vi "FPGA_target_reset_memory.vi"(0 "mem_addr_in":u32) -> (14 "mem_addr_out":u32)   [LabVIEW 2014]
doc: "Clears memory from specified index."
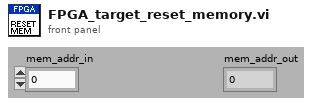
[diagram p1: front panel]
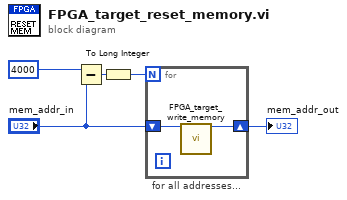
[diagram p0: block diagram]
diagram:
  n1 = Subtract(x=u32 4000, y="mem_addr_in") -> (x-y=w3:u32)
  n2 = To Long Integer(number=w3) -> (32bit integer=w4:i32)
  n3 = for "for all addresses..." {
    N: w4 -> [_]
    shift-right: [w6] -> w1
    shift-left: "mem_addr_in" -> [w7]
    n4 = call "FPGA_target_write_memory.vi"("mem_addr_in"=w7) -> ("mem_addr_out"=w6:u32)  [unwired: 18 in]
  }
  "mem_addr_out" <- w1
